vi "Kalman_Filter_Getter.vi"(8 "error in (no error)":errorcluster, 11 "Kalman_Filter in":refnum<class "Kalman_Filter.lvclass">) -> (0 "error out":errorcluster, 1 "P process cov":dbl[][](array[numeric]), 2 "State":dbl[][](array[numeric]), 3 "Kalman_Filter out":refnum<class "Kalman_Filter.lvclass">)   [LabVIEW 2021, in "Kalman_Filter.lvclass"]
uses:
  Kalman_Filter.lvclass
  Kalman_Filter.lvclass/Kalman_Filter.ctl
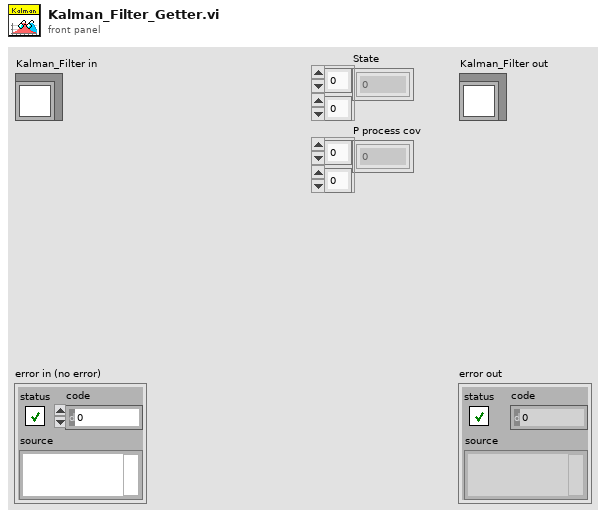
[diagram p1: front panel]
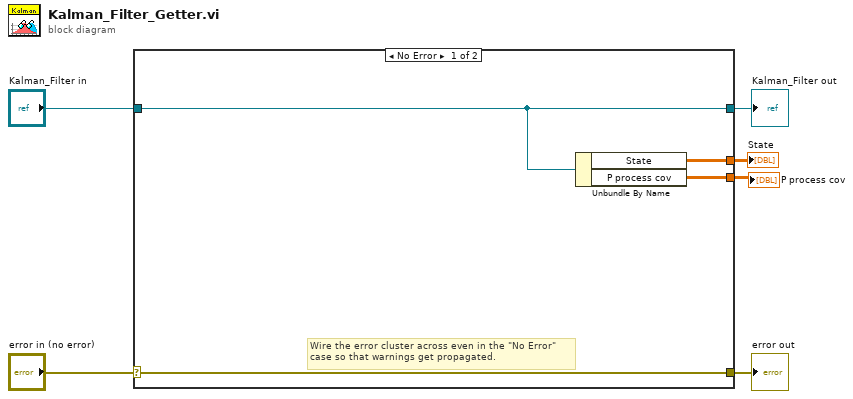
[diagram p0: block diagram]
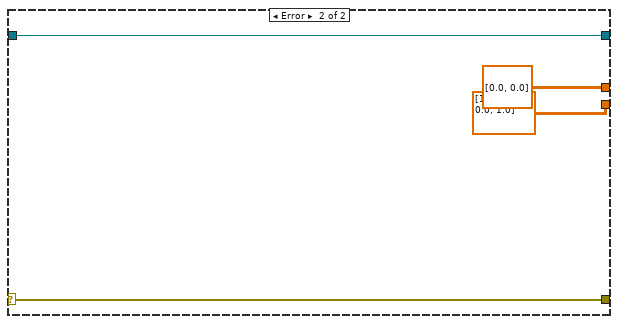
[diagram p2: hidden frame]
diagram:
  n1 = case shown="No Error" "error in (no error)" {
    selector: "error in (no error)" -> [w10 w14]
    tunnel: [w10 w14] -> w5
    tunnel: [w9 w13] -> w3
    tunnel: "Kalman_Filter in" -> [w9 w13]
    tunnel: [w8 dbl[][] [[0.0], [0.0]] ("State")] -> w2
    tunnel: [w7 dbl[][] [[1.0, 0.0], [0.0, 1.0]] ("P process cov")] -> w1
    frame No Error {
      # "Wire the error cluster across even in the \"No Error\"\ncase so that warnings get propagated."
      n2 = Unbundle By Name(w9) -> ("State"=w8:dbl[][], "P process cov"=w7:dbl[][])
    }
    frame Error {
    }
  }
  "error out" <- w5
  "Kalman_Filter out" <- w3
  "State" <- w2
  "P process cov" <- w1
